vi "Test Pdash Style.vi"() -> ()   [LabVIEW 2020, in "Panther Dashboard.lvlib"]
uses:
  Panther Dashboard.lvlib
  Controls/Listbox.ctl
  Controls/MulticolumListbox.ctl
  <vilib>/National Instruments/Tree Map/API/List Roots.vi
  <vilib>/National Instruments/Tree Map/Utility/Into Tree Control Items.vi
  <vilib>/National Instruments/Tree Map/Tree Map.lvlib
panel:
  out "String Out":string
  in  "Button":bool
  in  "String":string="test text"
  in  "Tree Control":string(tree)
  in  "Boolean 2":bool
  in  "Blank Button":bool
  in  "OK Button":bool
  in  "Boolean":bool
  in  "Button 2":bool
  in  "Tank":dbl(slide) scale=0.0..10.0
  out "Numeric 2":dbl
  in  "Numeric":dbl
  in  "Listbox":T1
  in  "Results Listbox":T2
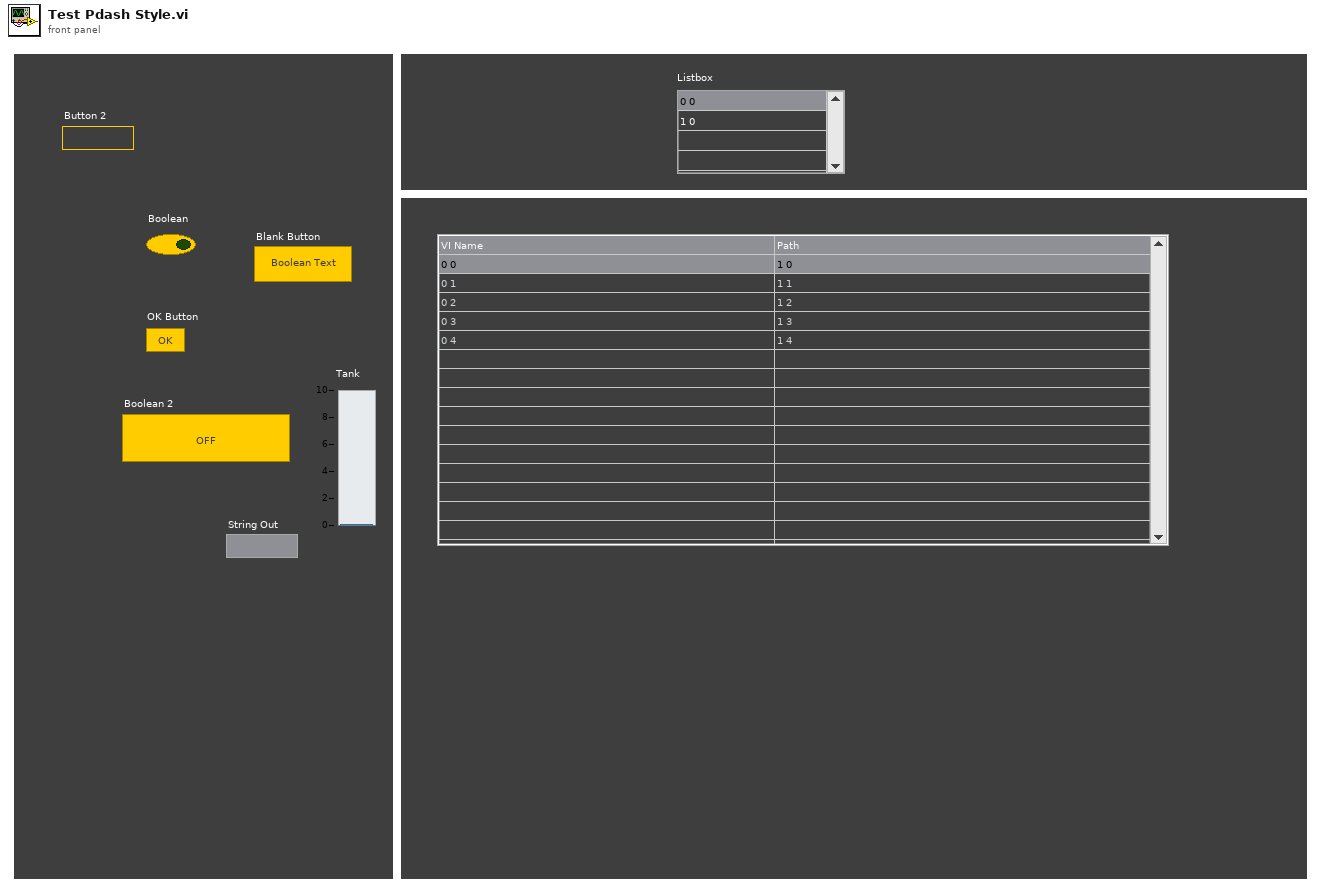
[diagram p1: front panel]
types:
  T1 = typedef "Listbox.ctl" = i32
  T2 = typedef "MulticolumListbox.ctl" = i32
  T3 = typedef "Tree Map.lvlib/Tree Map Data.ctl" = map{string, cluster{"Child Paths Set":set{string}, "Name":string, "Data":string, "Attributes":map{string, string}}}
  T4 = cluster{"Left Cell String":string, "Child Text":string[], "Child Tag":string, "Item Indent":i32, "Child Only?":bool, "Glyph Index":i32}[]
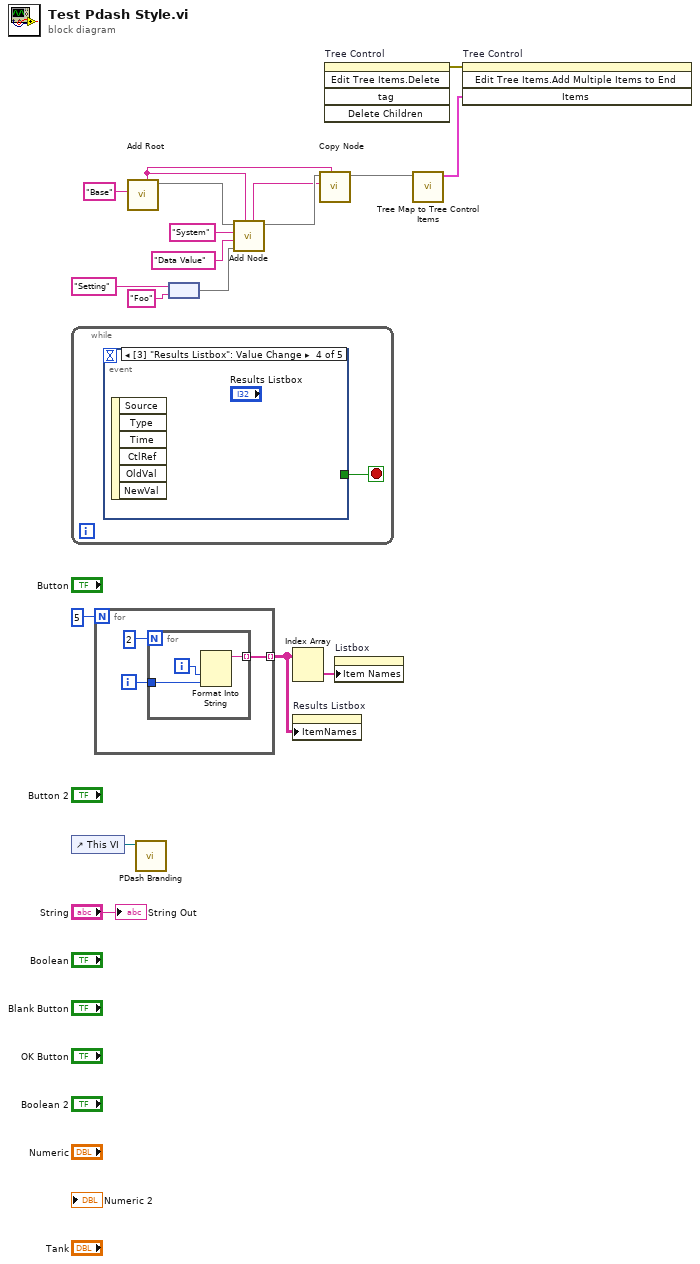
[diagram p0: block diagram]
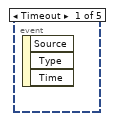
[diagram p2: hidden frame]
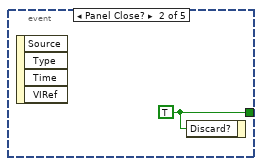
[diagram p3: hidden frame]
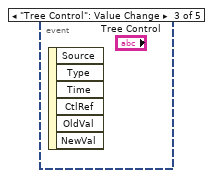
[diagram p4: hidden frame]
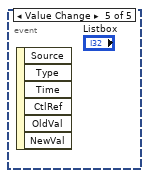
[diagram p5: hidden frame]
diagram:
  n1 = while {
    stop <- w19 stop-if-true
    n2 = event shown="[3] \"Results Listbox\": Value Change" {
      selector: _ -> [_ _ _ _ _]
      dyn-events: _ -> [_ _ _ _ _]
      timeout: _ -> [_ _ _ _ _]
      tunnel: [_ w20 _ _ _] -> w19
      event Timeout {
        n3 = event-data() -> ()  [unwired: 1 in, 3 out]
      }
      event Panel Close? {
        w20 = TRUE ("Discard?")
        n4 = event-data() -> ()  [unwired: 1 in, 4 out]
        n5 = event-data("Discard?"=w20) -> ()  [unwired: 1 in, 1 out]
      }
      event "Tree Control": Value Change {
        n6 = event-data() -> ()  [unwired: 1 in, 6 out]
      }
      event Value Change {
        n7 = event-data() -> ()  [unwired: 1 in, 6 out]
      }
      event Value Change {
        n8 = event-data() -> ()  [unwired: 1 in, 6 out]
      }
    }
  }
  n9 = control-ref of="This VI"() -> (w16:refnum<vi>)
  n10 = for {
    N: 5 -> [_]
    tunnel: [w22] -> w2 mode=indexing
    i -> [w23]
    n11 = for {
      N: 2 -> [_]
      tunnel: w23 -> [w25]
      tunnel: [w24] -> w22 mode=indexing
      i -> [w26]
      n12 = Format Into String(w26, w25) -> (resulting string=w24:string)  [unwired: 3 in, 1 out]
    }
  }
  n13 = call <vilib>:"Add Root.vi"("New Root Name"="Base") -> ("Tree Map Out"=w14:T3, "Root Path"=w6:string)  [unwired: 9 in]
  n14 = call "PDash Branding.vi"("This VI"=w16) -> ()  [unwired: 11 in]
  n15 = node("Setting" ("New Root Name"), "Foo" ("New Root Name")) -> (w11:map{string, string})
  n16 = call <vilib>:"Add Node.vi"("Parent Path"=w6, "Attributes"=w11, "Data"="Data Value" ("New Root Name"), "New Node Name"="System" ("New Root Name"), "Tree Map In"=w14) -> ("Tree Map Out"=w5:T3, "New Node Path"=w4:string)  [unwired: 4 in, 1 out]
  n17 = Index Array(array=w2) -> (element=w1:string[])  [unwired: 2 in]
  n18 = property on="Results Listbox" class="MCListbox (strict)"("ItemNames"=w2) -> ()  [unwired: 2 in, 2 out]
  n19 = call <vilib>:"Copy Node.vi"("New Parent Path in Target"=w6, "Node Path in Source"=w4, "Target Tree Map In"=w5) -> ("Target Tree Map Out"=w7:T3)  [unwired: 6 in, 2 out]
  n20 = invoke on="Tree Control" class="Tree (strict)" method="Edit Tree Items.Delete"() -> (error out=w18:errorcluster)  [unwired: 5 in, 4 out]
  n21 = property on="Listbox" class="LstBox (strict)"("Item Names"=w1) -> ()  [unwired: 2 in, 2 out]
  n22 = call <vilib>:"Tree Map to Tree Control Items.vi"("Tree Map In"=w7) -> ("Tree Control Items"=w8:T4)  [unwired: 10 in]
  n23 = invoke on="Tree Control" class="Tree (strict)" method="Edit Tree Items.Add Multiple Items to End"(error in=w18, "Items"=w8) -> ()  [unwired: 2 in, 4 out]
  "String Out" <- "String"
